vi "PendulumLoop.Outputs.ci.vi"() -> ()   [LabVIEW 2017, in "PendulumLoop.lvlib"]
uses:
  PendulumLoop.lvlib
panel:
  in  "Pendulum Angle":dbl
  in  "Cart X":dbl
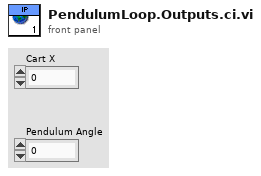
[diagram p1: front panel]
diagram:
